vi "Stop.vi"() -> ()   [LabVIEW 2013]
panel:
  in  "stop":bool
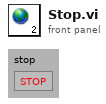
[diagram p1: front panel]
diagram:
